vi "Subtractor1.vi"() -> (8 "Subtractor1":refnum<class "Subtractor1.lvclass">)   [LabVIEW 2017, in "Subtractor1.lvclass"]
uses:
  Subtractor1.lvclass
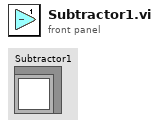
[diagram p1: front panel]
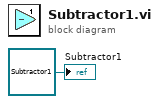
[diagram p0: block diagram]
diagram:
  "Subtractor1" <- refnum<class "Subtractor1.lvclass"> refnum ("Subtractor1.lvclass")
